vi "Get Commd.vi"(8 "error in (no error)":errorcluster, 11 "Channel in":refnum<class "Channel.lvclass">) -> (0 "error out":errorcluster, 3 "Channel out":refnum<class "Channel.lvclass">)   [LabVIEW 2018, in "Channel.lvclass"]
uses:
  Channel.lvclass
  Channel.lvclass/Channel.ctl
  RxTx/RxTx.lvclass
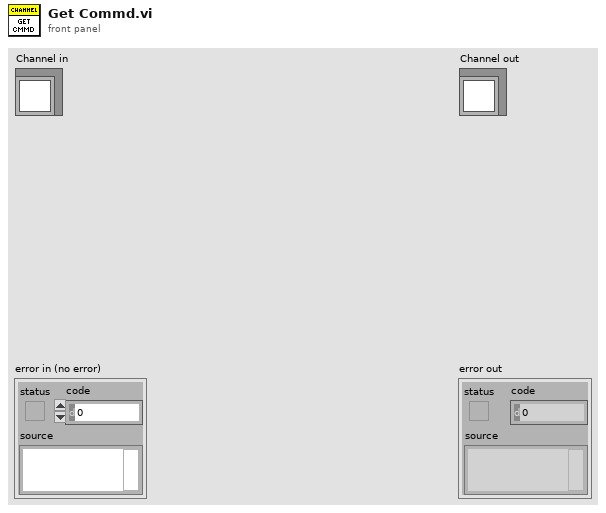
[diagram p1: front panel]
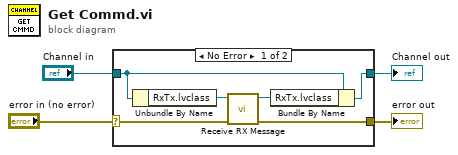
[diagram p0: block diagram]
diagram:
  n1 = case shown="No Error" "error in (no error)" {
    selector: "error in (no error)" -> [w5 w12]
    tunnel: [w6 w12] -> w3
    tunnel: [w9 w11] -> w1
    tunnel: "Channel in" -> [w10 w11]
    frame No Error {
      n2 = Unbundle By Name(w10) -> ("RxTx.lvclass"=w7:refnum<class "RxTx.lvclass">)
      n3 = call "Receive RX Message.vi"("error in (no error)"=w5, "RxTx in"=w7) -> ("error out"=w6:errorcluster, "RxTx out"=w8:refnum<class "RxTx.lvclass">)  [unwired: 8 in]
      n4 = Bundle By Name(cluster=w10, "RxTx.lvclass"=w8) -> (w9:refnum<class "Channel.lvclass">)
    }
    frame Error {
    }
  }
  "error out" <- w3
  "Channel out" <- w1
